vi "löschen.vi"(6 "F_max in %":sgl, 9 "Eingabetabelle":T2, 10 "Polynom-Ordnung":i32, 11 "Protokoll-Info":T3) -> (3 "Polynomanpassung":T1 {"Polynomkoeff." format="%#_10g"})   [LabVIEW 2015]
uses:
  Linearisierung/AutoLin Protokoll-Info.ctl
  Eingabetabelle.ctl
  Linearisierung/AutoLin Lin-Polynom.ctl
  Linearisierung/Aktionen Lin Daten aufarbeiten.ctl
  <vilib>/Analysis/6fits.llb/Curve Fitting Criteria.ctl
  Linearisierung/Linearisierung.lvlib
  <vilib>/Analysis/NI_AALPro.lvlib
  Linearisierung/AutoLin Protokoll/AutoLin Protokoll.lvlib
  Neue Linearisierung.lvlib
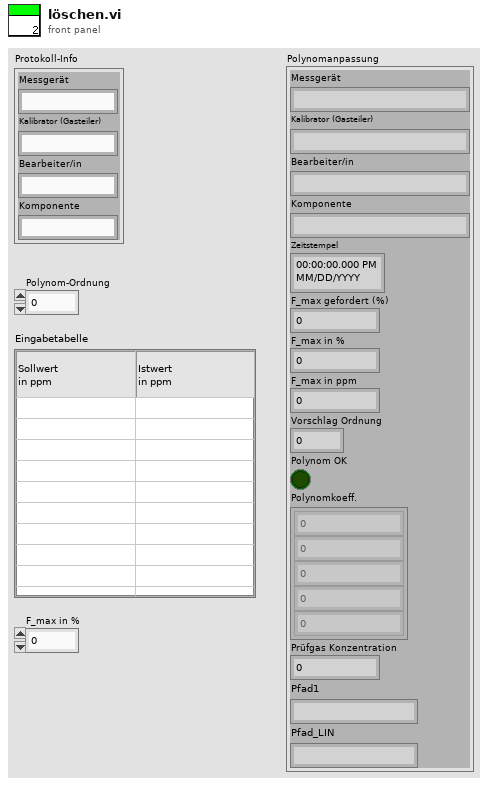
[diagram p1: front panel]
types:
  T1 = typedef "Linearisierung.lvlib/AutoLin Lin-Polynom.ctl" = cluster{"Messgerät":string, "Kalibrator (Gasteiler)":string, "Bearbeiter/in":string, "Komponente":string, "Zeitstempel":timestamp, "F_max gefordert (%)":sgl, "F_max in %":sgl, "F_max in ppm":sgl, "Vorschlag Ordnung":i32, "Polynom OK":bool, "Polynomkoeff.":sgl[], "Prüfgas Konzentration":sgl, "Pfad1":string, "Pfad_LIN":string}
  T2 = typedef "Neue Linearisierung.lvlib/Eingabetabelle.ctl" = string[][]
  T3 = typedef "Linearisierung.lvlib/AutoLin Protokoll-Info.ctl" = cluster{"Messgerät":string, "Kalibrator (Gasteiler)":string, "Bearbeiter/in":string, "Komponente":string}
  T4 = typedef "Linearisierung.lvlib/Aktionen Lin Daten aufarbeiten.ctl" = enum16{"lesen", "Rohdaten", "Protkolldaten", "Sollwerte", "Istwerte", "Schwankung", "Prtk. speichern", "Prtk. laden", "laden aktiv"}
  T5 = typedef "NI_AALPro.lvlib/Curve Fitting Criteria.ctl" = u16
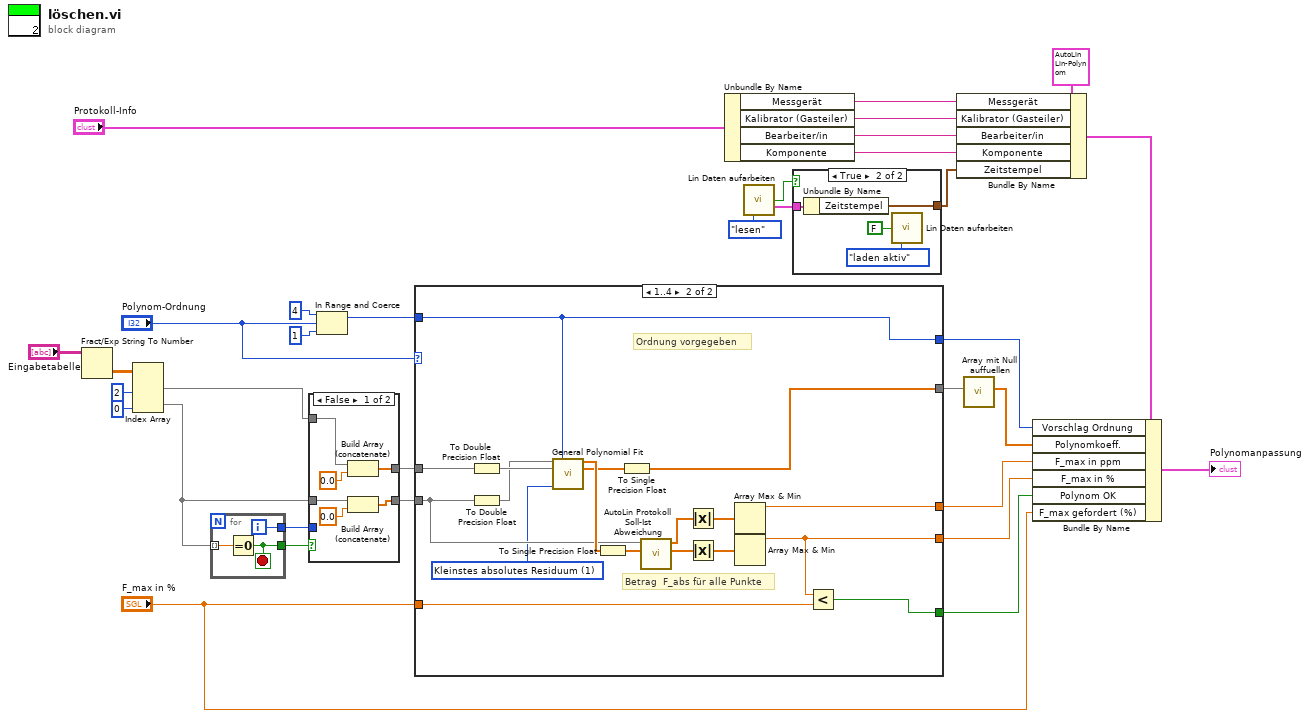
[diagram p0: block diagram]
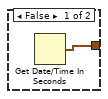
[diagram p2: hidden frame]
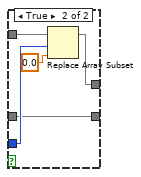
[diagram p3: hidden frame]
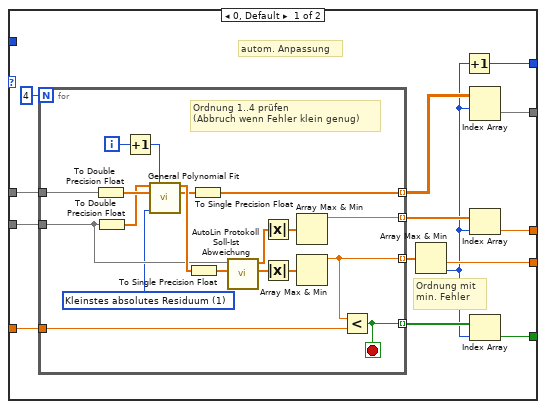
[diagram p4: hidden frame]
diagram:
  n1 = Fract/Exp String To Number(string="Eingabetabelle") -> (number=w28:dbl[][])  [unwired: 3 in, 1 out]
  n2 = Index Array(array=w28, index (col) #1=2 ("Deaktivierter Index (Spalte)"), index (col) #2=0 ("Index (Spalte)")) -> (element #1=w30:dbl[], element #2=w32:dbl[])  [unwired: 2 in]
  n3 = for {
    tunnel: w32 -> [w36] mode=indexing
    tunnel: [w35] -> w21
    tunnel: [w34] -> w20
    i -> [w34]
    stop <- w35 stop-if-true
    n4 = Equal To 0?(x=w36) -> (x = 0?=w35:bool)
  }
  n5 = case shown="False" w21 {
    tunnel: w30 -> [w42 w47]
    tunnel: w32 -> [w37 w44]
    tunnel: [w41 w46] -> w18
    tunnel: [w38 w44] -> w19
    tunnel: w20 -> [_ w45]
    frame False {
      n6 = Build Array (concatenate)(w42, sgl 0.0) -> (w41:dbl[])
      n7 = Build Array (concatenate)(w37, sgl 0.0) -> (w38:dbl[])
    }
    frame True {
      n8 = Replace Array Subset(array=w47, new element=sgl 0.0 ("Neues Element/Teil-Array"), index=w45) -> (w46:dbl[])
    }
  }
  n9 = In Range and Coerce(upper limit=4 ("Obergrenze"), x="Polynom-Ordnung", lower limit=1 ("Untergrenze")) -> (coerced(x)=w13:i32)  [unwired: 1 out]
  n10 = case shown="1..4" "Polynom-Ordnung" {
    tunnel: w18 -> [w61 w93]
    tunnel: w19 -> [w60 w87]
    tunnel: w13 -> [_ w94]
    tunnel: "F_max in %" -> [w58 w98]
    tunnel: [w55 w88] -> w22
    tunnel: [w57 w96] -> w17
    tunnel: [w52 w95] -> w2
    tunnel: [w54 w94] -> w16
    tunnel: [w48 w83] -> w15
    frame 0, Default {
      # "Ordnung mit\nmin. Fehler"
      # "autom. Anpassung"
      n11 = for {
        N: 4 -> [_]
        tunnel: w61 -> [w74]
        tunnel: w60 -> [w67]
        tunnel: [w70] -> w56 mode=indexing
        tunnel: w58 -> [w79]
        tunnel: [w75] -> w51 mode=indexing
        tunnel: [w76] -> w53 mode=indexing
        tunnel: [w63] -> w50 mode=indexing
        i -> [w80]
        stop <- w76 stop-if-true
        w62 = T5 1 items=["Kleinstes Quadrat", "Kleinstes absolutes Residuum", "Biquadrat"] ("method")
        # "Ordnung 1..4 prüfen\n(Abbruch wenn Fehler klein genug)"
        n12 = To Double Precision Float(number=w74) -> (double precision float=w73:dbl[])
        n13 = To Double Precision Float(number=w67) -> (double precision float=w72:dbl[])
        n14 = Increment(x=w80) -> (x+1=w77:i32)
        n15 = call <vilib>:"General Polynomial Fit.vi"("Y"=w72, "polynomial order"=w77, "X"=w73, "method"=w62) -> ("Best Polynomial Fit"=w71:dbl[], "Polynomial Coefficients"=w69:dbl[])  [unwired: 8 in, 2 out]
        n16 = To Single Precision Float(number=w71) -> (single precision float=w68:sgl[])
        n17 = To Single Precision Float(number=w69) -> (single precision float=w70:sgl[])
        n18 = call "AutoLin Protokoll Soll-Ist Abweichung.vi"("Istwerte (ppm)"=w68, "Sollwerte (ppm)"=w67) -> ("% vom Sollwert"=w66:sgl[], "abs. Fehler (ppm)"=w65:sgl[])  [unwired: 7 in, 1 out]
        n19 = Absolute Value(x=w65) -> (abs(x)=w64:sgl[])
        n20 = Absolute Value(x=w66) -> (abs(x)=w78:sgl[])
        n21 = Array Max & Min(array=w64) -> (max value=w63:sgl)  [unwired: 3 out]
        n22 = Array Max & Min(array=w78) -> (max value=w75:sgl)  [unwired: 3 out]
        n23 = Less?(x=w75, y=w79) -> (x < y?=w76:bool)
      }
      n24 = Array Max & Min(array=w51) -> (min value=w57:sgl, min index (indices)=w49:i32)  [unwired: 2 out]
      n25 = Increment(x=w49) -> (x+1=w54:i32)
      n26 = Index Array(array=w56, index (row)=w49) -> (element=w55:sgl[])  [unwired: 1 in]
      n27 = Index Array(array=w50, index=w49) -> (element=w48:sgl)
      n28 = Index Array(array=w53, index=w49) -> (element=w52:bool)
    }
    frame 1..4 {
      w81 = T5 1 items=["Kleinstes Quadrat", "Kleinstes absolutes Residuum", "Biquadrat"] ("method")
      # "Betrag  F_abs für alle Punkte"
      # "Ordnung vorgegeben"
      n29 = To Double Precision Float(number=w93) -> (double precision float=w92:dbl[])
      n30 = To Double Precision Float(number=w87) -> (double precision float=w91:dbl[])
      n31 = call <vilib>:"General Polynomial Fit.vi"("Y"=w91, "polynomial order"=w94, "X"=w92, "method"=w81) -> ("Best Polynomial Fit"=w90:dbl[], "Polynomial Coefficients"=w89:dbl[])  [unwired: 8 in, 2 out]
      n32 = To Single Precision Float(number=w90) -> (single precision float=w86:sgl[])
      n33 = To Single Precision Float(number=w89) -> (single precision float=w88:sgl[])
      n34 = call "AutoLin Protokoll Soll-Ist Abweichung.vi"("Istwerte (ppm)"=w86, "Sollwerte (ppm)"=w87) -> ("% vom Sollwert"=w85:sgl[], "abs. Fehler (ppm)"=w82:sgl[])  [unwired: 7 in, 1 out]
      n35 = Absolute Value(x=w82) -> (abs(x)=w84:sgl[])
      n36 = Absolute Value(x=w85) -> (abs(x)=w97:sgl[])
      n37 = Array Max & Min(array=w84) -> (max value=w83:sgl)  [unwired: 3 out]
      n38 = Array Max & Min(array=w97) -> (max value=w96:sgl)  [unwired: 3 out]
      n39 = Less?(x=w96, y=w98) -> (x < y?=w95:bool)
    }
  }
  n40 = Unbundle By Name("Protokoll-Info") -> ("Messgerät"=w5:string, "Kalibrator (Gasteiler)"=w6:string, "Bearbeiter/in"=w7:string, "Komponente"=w10:string)
  n41 = call "Lin Daten aufarbeiten.vi"("Aktionen"=Aktionen_Lin_Daten_aufarbeiten."lesen") -> ("Laden aktiv?"=w25:bool, "Lin-Polynom"=w26:T1)  [unwired: 10 in, 3 out]
  n42 = case shown="True" w25 {
    tunnel: [w99 w101] -> w9
    tunnel: w26 -> [_ w102]
    frame False {
      n43 = Get Date/Time In Seconds() -> (seconds since 1Jan1904=w99:timestamp)
    }
    frame True {
      n44 = Unbundle By Name(w102) -> ("Zeitstempel"=w101:timestamp)
      n45 = call "Lin Daten aufarbeiten.vi"("Laden aktiv?"=FALSE, "Aktionen"=Aktionen_Lin_Daten_aufarbeiten."laden aktiv") -> ()  [unwired: 9 in, 5 out]
    }
  }
  n46 = Bundle By Name(cluster=T1 {"Messgerät"="", "Kalibrator (Gasteiler)"="", "Bearbeiter/in"="", "Komponente"="", "Zeitstempel"=timestamp(0 s since 1904-01-01), "F_max gefordert (%)"=0.0, "F_max in %"=0.0, "F_max in ppm"=0.0, "Vorschlag Ordnung"=0, "Polynom OK"=FALSE, "Polynomkoeff."=[], "Prüfgas Konzentration"=0.0, "Pfad1"="", "Pfad_LIN"=""} ("Polynomanpassung"), "Messgerät"=w5, "Kalibrator (Gasteiler)"=w6, "Bearbeiter/in"=w7, "Komponente"=w10, "Zeitstempel"=w9) -> (w8:T1)
  n47 = call "Array mit Null auffuellen.vi"("Array"=w22) -> ("Array 2"=w23:sgl[])  [unwired: 10 in]
  n48 = Bundle By Name(cluster=w8, "Vorschlag Ordnung"=w16, "Polynomkoeff."=w23, "F_max in ppm"=w15, "F_max in %"=w17, "Polynom OK"=w2, "F_max gefordert (%)"="F_max in %") -> (→"Polynomanpassung":T1)
